vi "clipconfv2.vi"() -> ()   [LabVIEW 2009]
uses:
  <vilib>/Utility/NIReport.llb/NI_report.lvclass
  <instrlib>/Agilent 81150/Agilent 81150.lvlib
  <vilib>/Analysis/NI_AALBase.lvlib
panel:
  out "mean value 2":dbl=711.9915188935893
  in  "Copnf value":i32[](array[numeric])=[400, 380, 350, 320, 300, 280, 250, 220, 200, 180, 150, 120, 100]
  out "Numeric 3":i32
  out "error out":errorcluster
  out "Quantity bucle":i32=62
  out "mean value":dbl=711.9915188935893
  in  "Voltages comprobation":dbl[](array[numeric])=[0.05, 0.1, 0.2, 0.3, 0.35, 0.4, 0.45, 0.5, 0.55, 0.6, 0.7, 0.8, 0.9, 1.0, 1.2, 1.4, 1.6, 1.8, 2.0, 2.2, 2.5]
  out "Vatt":i32[](array[numeric])=[2200, 2200, 2200, 2200, 2200, 2200]
  out "Vclip":i32[](array[numeric])=[415, 417, 409, 455, 424, 466]
  in  "Vclip end":i32[](array[numeric])
  in  "Vatt end":i32[](array[numeric])
  in  "Vatt ini":i32[](array[numeric])=[4095, 4095, 4095, 4095, 4095, 4095, 4095]
  in  "Vclip ini":i32[](array[numeric])=[0, 0, 0, 0, 0, 0, 0]
  out "Vclip end":i32[](array[numeric])
  out "Vatt end":i32[](array[numeric])
  out "Numeric 2":i32
  out "Numeric":i32
  in  "Channels":i32[](array[numeric])=[0, 1, 2, 3, 4, 5, 6]
  in  "Cycles Burst":i32=10000
  out "IPR_Address":i32=23
  out "L1 Address":i32=17
  in  "L1 version":bool
  in  "Instrument VISA in":T1={"AWG VISA"="81160A", "Oscilloscope  VISA "="DSO80204B", "Integration Board IP"="172.16.7.43", "connection ID"=refnum, "report out"=refnum, "report file path"=path "D:/CTA/Data_test"}
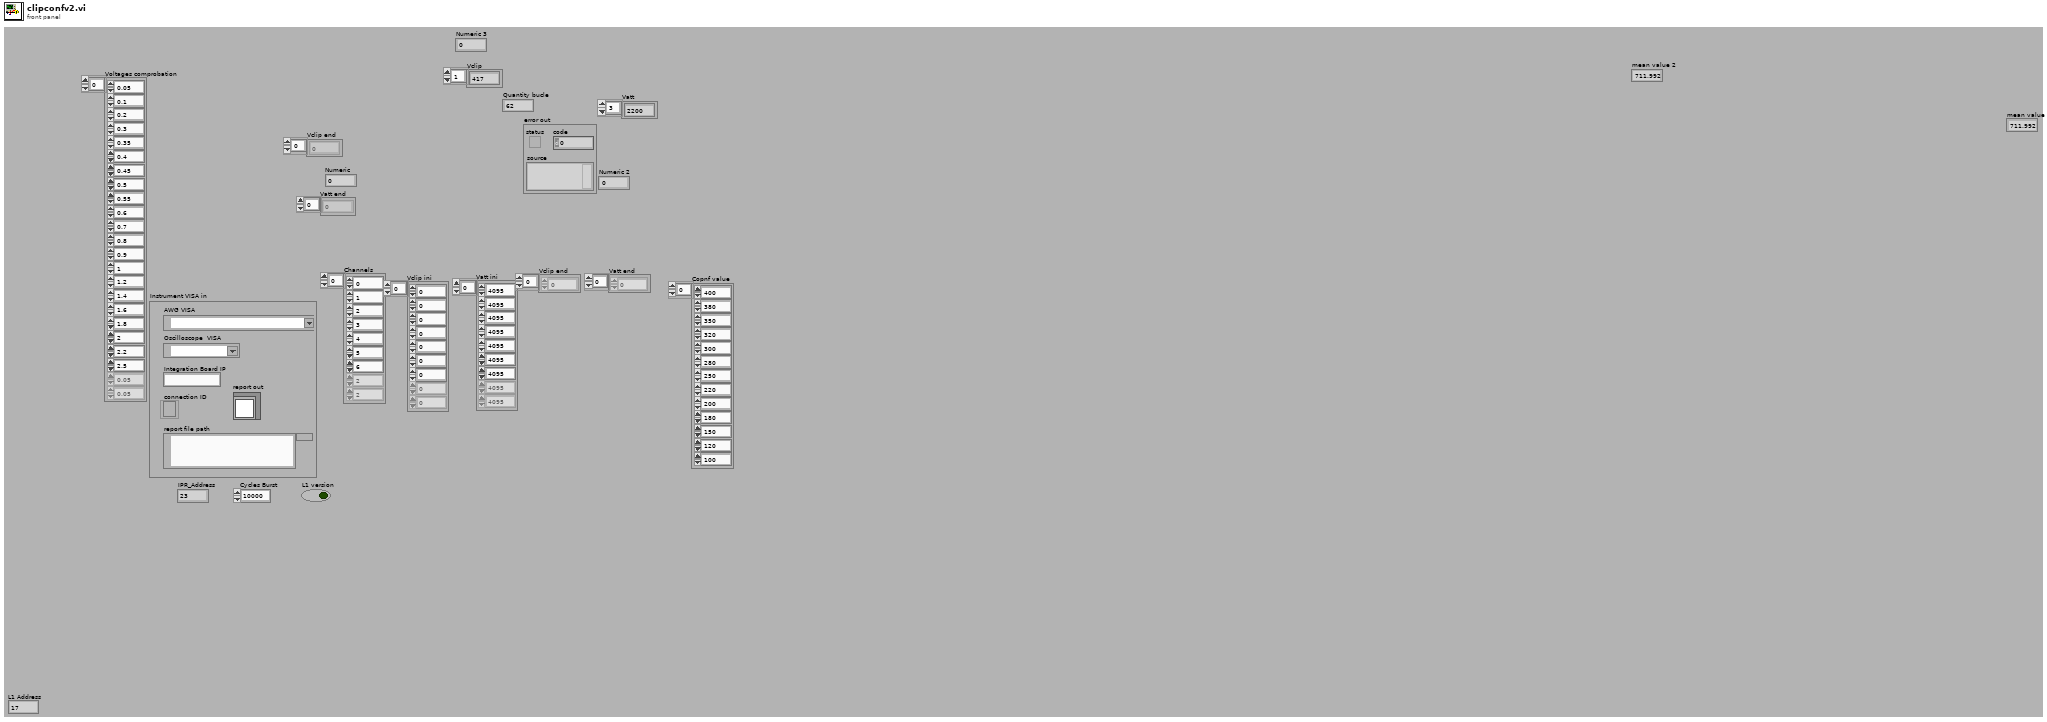
[diagram p1: front panel]
types:
  T1 = cluster{"AWG VISA":refnum<visa-resource-name>, "Oscilloscope  VISA ":refnum<visa-resource-name>, "Integration Board IP":string, "connection ID":refnum<k5>, "report out":refnum<class "NI_report.lvclass">, "report file path":path}
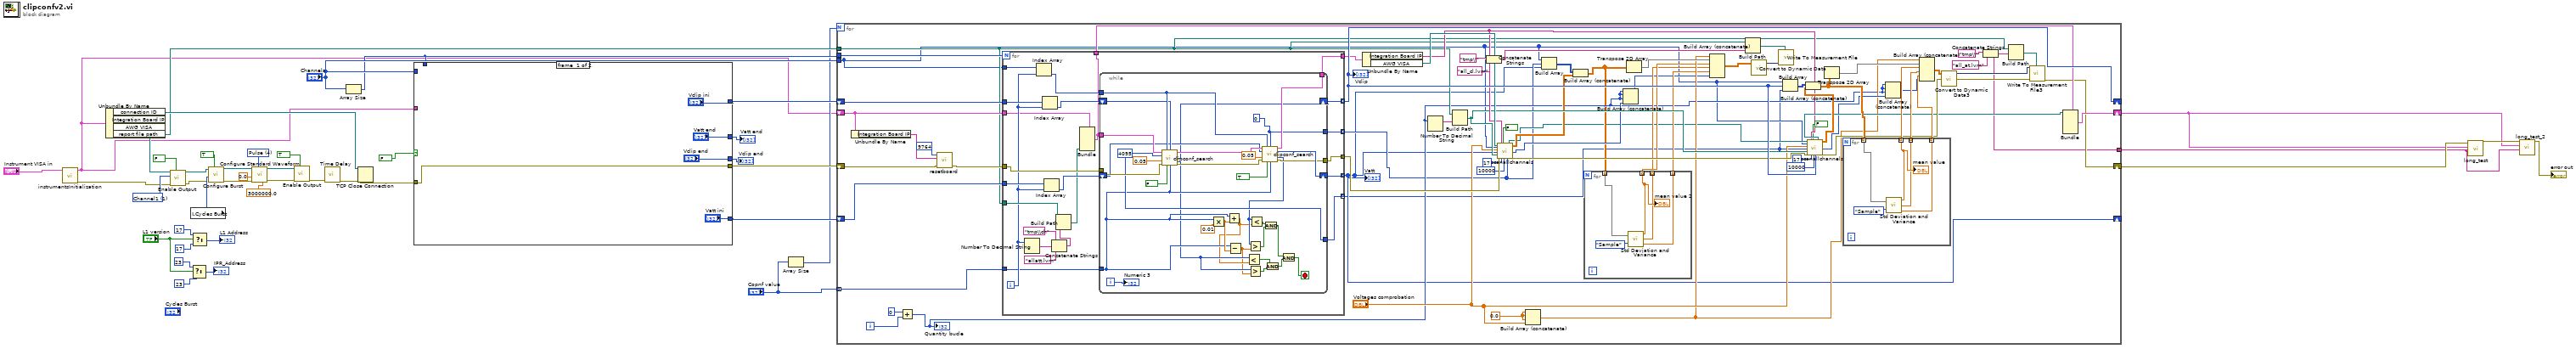
[diagram p0: block diagram]
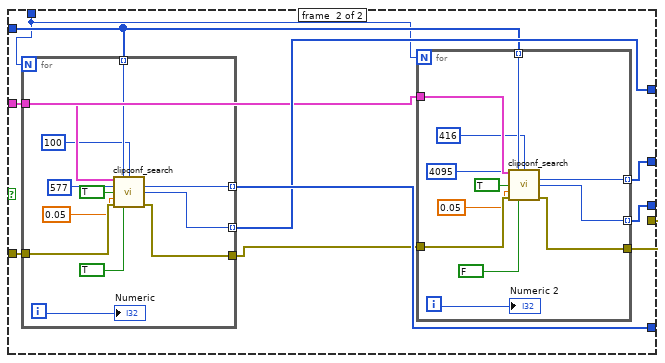
[diagram p2: hidden frame]
diagram:
  w37 = u16 4 items=["Sine", "Square", "Ramp Up", "Ramp Down", "Pulse", "Noise", "DC"] ("Waveform (0: Sine)")
  w43 = u16 1 items=["Channel1"=1, "Channel2"=2] ("Channel (1: Channel1)")
  n1 = call "instrumentsInitialization.vi"("Instrument VISA in"="Instrument VISA in") -> ("error out"=w22:errorcluster, "Instrument VISA out"=w2:T1)  [unwired: 9 in]
  n2 = Unbundle By Name(w2) -> ("connection ID"=w25:refnum<k5>, "AWG VISA"=w38:refnum<visa-resource-name>, "report file path"=w13:path)  [unwired: 1 out]
  n3 = call <instrlib>:"Enable Output.vi"("Enable Output (T: Enable)"=FALSE, "error in (no error)"=w22, "Channel (1: Channel1)"=w43, "VISA resource name"=w38) -> ("error out"=w24:errorcluster, "VISA resource name out"=w23:refnum<visa-resource-name>)  [unwired: 6 in]
  n4 = local read "Cycles Burst"() -> (w26:i32)
  n5 = Select(t=23 ("Address"), s="L1 version", f=23 ("Address")) -> (s? t:f=→"IPR_Address":i32)
  n6 = Select(t=17 ("Address"), s="L1 version", f=17 ("Address")) -> (s? t:f=→"L1 Address":i32)
  n7 = call <instrlib>:"Configure Burst.vi"("Enable Burst (F: Disable)"=TRUE, "error in (no error)"=w24, "Burst Count (2)"=w26, "VISA resource name"=w23) -> ("error out"=w34:errorcluster, "VISA resource name out"=w35:refnum<visa-resource-name>)  [unwired: 6 in]
  n8 = call <instrlib>:"Configure Standard Waveform.vi"("Frequency (1000.0 Hz)"=3000000.0, "Waveform (0: Sine)"=w37, "error in (no error)"=w34, "Amplitude (1.0 Vpp)"=0.0, "VISA resource name"=w35) -> ("error out"=w33:errorcluster, "VISA resource name out"=w21:refnum<visa-resource-name>)  [unwired: 5 in]
  n9 = call <instrlib>:"Enable Output.vi"("Enable Output (T: Enable)"=TRUE, "error in (no error)"=w33, "VISA resource name"=w21) -> ("error out"=w14:errorcluster)  [unwired: 7 in, 1 out]
  n10 = call "Time Delay"("error in (no error)"=w14) -> ("error out"=w15:errorcluster)  [unwired: 10 in]
  n11 = Array Size(array="Channels") -> (size(s)=w12:i32)
  n12 = TCP Close Connection(connection ID=w25, error in (no error)=w15) -> (error out=w20:errorcluster)  [unwired: 1 in, 1 out]
  n13 = case shown="False" FALSE ("Boolean") {
    tunnel: w20 -> [w50 w60]
    tunnel: ["Vatt ini" w59] -> w19
    tunnel: ["Vclip ini" w58] -> w18
    tunnel: [w50 w56] -> w17
    tunnel: w2 -> [_ w55]
    tunnel: "Channels" -> [_ w54]
    tunnel: w12 -> [_ w53]
    tunnel: ["Vatt end" w52] -> w10
    tunnel: ["Vclip end" w51] -> w9
    frame #0 {
    }
    frame #1 {
      n14 = for {
        N: w53 -> [_]
        tunnel: w60 -> [w84]
        tunnel: [w83] -> w57
        tunnel: w55 -> [w82]
        tunnel: w54 -> [w81] mode=indexing
        tunnel: [w80] -> w59 mode=indexing
        tunnel: [w79] -> w58 mode=indexing
        i -> [w75]
        n15 = call "clipconf_search.vi"("input cluster"=w82, "Channel"=w81, "vclip"=100, "Vatt init"=577, "Boolean"=TRUE, "Voltage value"=0.05, "error out 2"=w84, "Att/clip"=TRUE) -> ("Vatt init"=w80:i32, "vclip"=w79:i32, "error out"=w83:errorcluster)  [unwired: 3 in, 2 out]
        "Numeric" <- w75
      }
      n16 = for {
        N: w53 -> [_]
        tunnel: w57 -> [w72]
        tunnel: [w71] -> w56
        tunnel: w55 -> [w70]
        tunnel: w54 -> [w69] mode=indexing
        tunnel: [w68] -> w52 mode=indexing
        tunnel: [w67] -> w51 mode=indexing
        i -> [w63]
        n17 = call "clipconf_search.vi"("input cluster"=w70, "Channel"=w69, "vclip"=416, "Vatt init"=4095, "Boolean"=TRUE, "Voltage value"=0.05, "error out 2"=w72, "Att/clip"=FALSE) -> ("Vatt init"=w68:i32, "vclip"=w67:i32, "error out"=w71:errorcluster)  [unwired: 3 in, 2 out]
        "Numeric 2" <- w63
      }
    }
  }
  "Vatt end" <- w10
  "Vclip end" <- w9
  n18 = Array Size(array="Copnf value") -> (size(s)=w3:i32)
  n19 = for {
    N: w3 -> [_]
    tunnel: "Channels" -> [w88]
    tunnel: w13 -> [w109]
    tunnel: w12 -> [w153]
    shift-right: [w86] -> _
    shift-left: w19 -> [w152]
    shift-right: [w146] -> _
    shift-left: w18 -> [w131]
    shift-right: [w144] -> w1
    shift-left: w2 -> [w134]
    shift-right: [w127] -> w8
    shift-left: w17 -> [w136]
    tunnel: [w126] -> w6
    tunnel: "Copnf value" -> [w122] mode=indexing
    i -> [w125]
    w106 = 0.0 ("element")
    n20 = Unbundle By Name(w134) -> ("Integration Board IP"=w133:string)
    n21 = Add(x=0, y=w125) -> (x+y=w98:i32)
    "Quantity bucle" <- w98
    n22 = call "resetboard.vi"("error in (no error)"=w136, "address"=w133, "remote port or service name"=u16 9764) -> ("error out"=w135:errorcluster)  [unwired: 7 in, 1 out]
    n23 = for {
      N: w153 -> [_]
      tunnel: w131 -> [w184]
      tunnel: w88 -> [w181]
      tunnel: w134 -> [w172]
      tunnel: w152 -> [w182]
      tunnel: w109 -> [w187]
      tunnel: [w175] -> w86 mode=indexing
      tunnel: w135 -> [w185]
      tunnel: [w177] -> w121
      tunnel: [w169] -> w146 mode=indexing
      tunnel: [w170] -> w145
      tunnel: [w168] -> w123
      tunnel: w122 -> [w167]
      tunnel: [w166] -> w87 mode=indexing
      tunnel: [w165] -> w85 mode=indexing
      i -> [w174]
      n24 = Number To Decimal String(number=w174) -> (decimal integer string=w186:string)  [unwired: 1 in]
      n25 = Index Array(array=w181, index=w174) -> (element=w176:i32)
      n26 = Index Array(array=w184, index=w174) -> (element=w173:i32)
      n27 = Index Array(array=w182, index=w174) -> (element=w183:i32)
      n28 = Concatenate Strings("tmp\\ch" ("name or relative path"), w186, "allatt.lvm" ("string")) -> (w180:string)
      n29 = Build Path(base path=w187, name or relative path=w180) -> (appended path=w171:path)
      n30 = Bundle(cluster=w172, "report file path"=w171) -> (w170:T1)  [unwired: 5 in]
      n31 = while {
        tunnel: w185 -> [w219]
        tunnel: [w208] -> w177
        tunnel: w176 -> [w213]
        shift-right: [w204] -> w169
        shift-left: w173 -> [w206]
        shift-right: [w212] -> w175
        shift-left: w183 -> [w205]
        tunnel: w170 -> [w217]
        tunnel: [w207] -> w168
        tunnel: w167 -> [w199]
        tunnel: [w203] -> w166
        tunnel: [w202] -> w165
        i -> [w211]
        stop <- w190 stop-if-true
        w203 = 0 ("vclip")
        w202 = 4095 ("Vatt init")
        n32 = call "clipconf_search.vi"("input cluster"=w217, "Channel"=w213, "vclip"=w206, "Vatt init"=w202, "Voltage value"=0.05, "error out 2"=w219, "Att/clip"=FALSE, "conf value"=w199) -> ("output cluster"=w215:T1, "vclip"=w204:i32, "L1 value"=w195:i32, "error out"=w216:errorcluster)  [unwired: 3 in, 1 out]
        n33 = Multiply(x=w199, y=0.01) -> (x*y=w200:dbl)
        n34 = Add(x=w199, y=w200) -> (x+y=w189:dbl)
        n35 = Subtract(x=w199, y=w200) -> (x-y=w188:dbl)
        n36 = Less?(x=w195, y=w189) -> (x < y?=w193:bool)
        n37 = Greater?(x=w195, y=w188) -> (0:w194:bool)
        n38 = call "clipconf_search.vi"("input cluster"=w215, "Channel"=w213, "vclip"=w203, "Vatt init"=w205, "Voltage value"=0.05, "error out 2"=w216, "Att/clip"=TRUE, "conf value"=w199) -> ("output cluster"=w207:T1, "Vatt init"=w212:i32, "L1 value"=w196:i32, "error out"=w208:errorcluster)  [unwired: 3 in, 1 out]
        n39 = Greater?(x=w196, y=w188) -> (0:w197:bool)
        n40 = Less?(x=w196, y=w189) -> (x < y?=w198:bool)
        n41 = And(x=w198, y=w197) -> (x .and. y?=w191:bool)
        n42 = And(x=w193, y=w194) -> (x .and. y?=w192:bool)
        n43 = And(x=w191, y=w192) -> (x .and. y?=w190:bool)
        "Numeric 3" <- w211
      }
    }
    "Vclip" <- w146
    "Vatt" <- w86
    n44 = Unbundle By Name(w123) -> ("Integration Board IP"=w119:string, "AWG VISA"=w120:refnum<visa-resource-name>)
    n45 = Number To Decimal String(number=w98) -> (decimal integer string=w115:string)  [unwired: 1 in]
    n46 = Build Path(base path=w109, name or relative path=w115) -> (appended path=w108:path)
    n47 = Concatenate Strings("tmp\\" ("name or relative path"), "all_cl.lvm" ("string")) -> (w110:string)
    n48 = call "scanallchannels.vi"("VISA resource name in"=w120, "nm ch"=w88, "Voltages values"="Voltages comprobation", "Init ch value"=w86, "base path"=w108, "error in"=w121, "Integration Board IP"=w119, "L1 Address"=17, "Save test data"=FALSE, "Ch burst"=10000, "vclip"=w87) -> ("VISA resource name out"=w93:refnum<visa-resource-name>, "L1  50%"=w104:dbl[][], "time"=w99:u32[], "error out"=w114:errorcluster)  [unwired: 4 in, 1 out]
    n49 = Build Array (concatenate)(w106, w106, w106, "Voltages comprobation") -> (w103:dbl[])
    n50 = Build Array(w88, w87, w86) -> (w89:i32[][])
    n51 = Build Array (concatenate)(w89, w104) -> (w94:dbl[][])
    n52 = for {
      tunnel: w94 -> [w159] mode=indexing
      tunnel: [w157] -> w102 mode=indexing
      tunnel: [w156] -> w101 mode=indexing
      tunnel: [w155] -> w100 mode=indexing
      n53 = call <vilib>:"Std Deviation and Variance.vi"("X"=w159, "Weighting (Sample)"=enum16{"Sample", "Population"}."Sample") -> ("mean"=w157:dbl, "standard deviation"=w156:dbl, "variance"=w155:dbl)
      "mean value 2" <- w157
    }
    n54 = Build Array (concatenate)(w98, w98, w98, w99) -> (w97:u32[])
    n55 = Transpose 2D Array(2D array=w94) -> (transposed array=w105:dbl[][])
    n56 = Build Array (concatenate)(w103, w105, w102, w101, w100, w97) -> (w96:dbl[][])
    n57 = Build Path(base path=w109, name or relative path=w110) -> (appended path=w111:path)
    n58 = call "Convert to Dynamic Data"("2D Array"=w96) -> ("Dynamic Data Type"=w95:dynamicdata)  [unwired: 3 in]
    n59 = call "Write To Measurement File"("Signals"=w95, "Filename"=w111) -> ()  [unwired: 15 in, 3 out]
    n60 = Build Array(w88, w146, w85) -> (w141:i32[][])
    n61 = call "scanallchannels.vi"("VISA resource name in"=w93, "nm ch"=w88, "Voltages values"="Voltages comprobation", "Init ch value"=w85, "base path"=w108, "error in"=w114, "Integration Board IP"=w119, "L1 Address"=17, "Save test data"=FALSE, "Ch burst"=10000, "vclip"=w146) -> ("VISA resource name out"=w137:refnum<visa-resource-name>, "L1  50%"=w142:dbl[][], "time"=w128:u32[], "error out"=w139:errorcluster)  [unwired: 4 in, 1 out]
    n62 = Build Array (concatenate)(w141, w142) -> (w140:dbl[][])
    n63 = Transpose 2D Array(2D array=w140) -> (transposed array=w150:dbl[][])
    n64 = for {
      tunnel: w140 -> [w164] mode=indexing
      tunnel: [w162] -> w149 mode=indexing
      tunnel: [w161] -> w148 mode=indexing
      tunnel: [w160] -> w147 mode=indexing
      n65 = call <vilib>:"Std Deviation and Variance.vi"("X"=w164, "Weighting (Sample)"=enum16{"Sample", "Population"}."Sample") -> ("mean"=w162:dbl, "standard deviation"=w161:dbl, "variance"=w160:dbl)
      "mean value" <- w162
    }
    n66 = Build Array (concatenate)(w98, w98, w98, w128) -> (w129:u32[])
    n67 = Build Array (concatenate)(w103, w150, w149, w148, w147, w129) -> (w143:dbl[][])
    n68 = call "Convert to Dynamic Data3"("2D Array"=w143) -> ("Dynamic Data Type"=w138:dynamicdata)  [unwired: 3 in]
    n69 = Concatenate Strings("tmp\\" ("name or relative path"), "all_at.lvm" ("string")) -> (w126:string)
    n70 = Build Path(base path=w109, name or relative path=w126) -> (appended path=w154:path)
    n71 = call "Write To Measurement File3"("Signals"=w138, "error in (no error)"=w139, "Filename"=w154) -> ("error out"=w127:errorcluster)  [unwired: 14 in, 2 out]
    n72 = Bundle(cluster=w145, "AWG VISA"=w137) -> (w144:T1)  [unwired: 5 in]
  }
  n73 = call "long_test.vi"("string"=w6, "Instrument VISA in"=w1, "error in (no error)"=w8) -> ("error out"=w7:errorcluster)  [unwired: 8 in]
  n74 = call "long_test_2.vi"("string"=w6, "Instrument VISA in"=w1, "error in (no error)"=w7) -> ("error out"=→"error out":errorcluster)  [unwired: 8 in]
